vi "Comments text in.vi"(0 "command text in":string[](array[string])=["N/A", "Magent PS", "N/A", "Set Field", "Set Field to 2.0000E+0 @ 0.0000T /min, no wait , extra 0 sec wait", "N/A", "N/A", "", "1", "0", "N/A", "2.000000", "0.000000", "N/A", "N/A", "N/A", "N/A", "N/A", "N/A", "N/A", "N/A", "N/A", "N/A", "N/A", "N/A", "N/A", "N/A", "N/A", "N/A", "N/A", "N/A", "N/A", "N/A", "N/A"]) -> (1 "commet string":string)   [LabVIEW 2020]
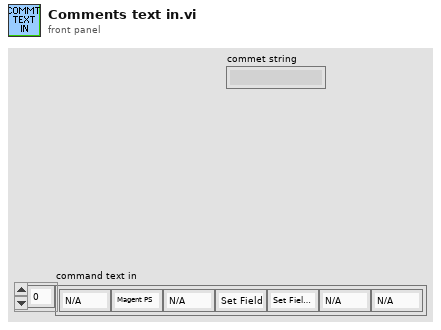
[diagram p1: front panel]
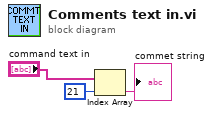
[diagram p0: block diagram]
diagram:
  n1 = Index Array(array="command text in", index=21) -> (element=→"commet string":string)
